vi "GetConfigFilePath.vi"(8 "error in (no error)":errorcluster caption="Fehler (Eingang, kein Fehler)", 10 "Main Vi Reference":refnum<vi>, 11 "ApplicationInititialisation Eingang":refnum<class "ApplicationInititialisation.lvclass"> caption="DNL_LabVIEW Object in") -> (0 "error out":errorcluster caption="Fehler (Ausgang)", 2 "Pfad":path, 3 "ApplicationInititialisation Ausgang":refnum<class "ApplicationInititialisation.lvclass"> caption="DNL_LabVIEW Object out")   [LabVIEW 2013, in "ApplicationInititialisation.lvclass"]
uses:
  ApplicationInititialisation.lvclass
panel:
  out "Ergebnis-String":string
  out "Applikation:Typ":T1(ring)
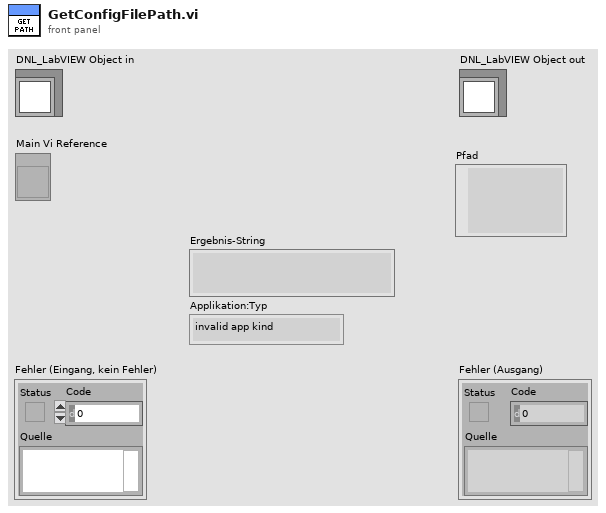
[diagram p1: front panel]
types:
  T1 = enum32{"invalid app kind", "Development System", "Run Time System", "Student Edition", "Embedded LabVIEW", "Evaluation", "Custom"}
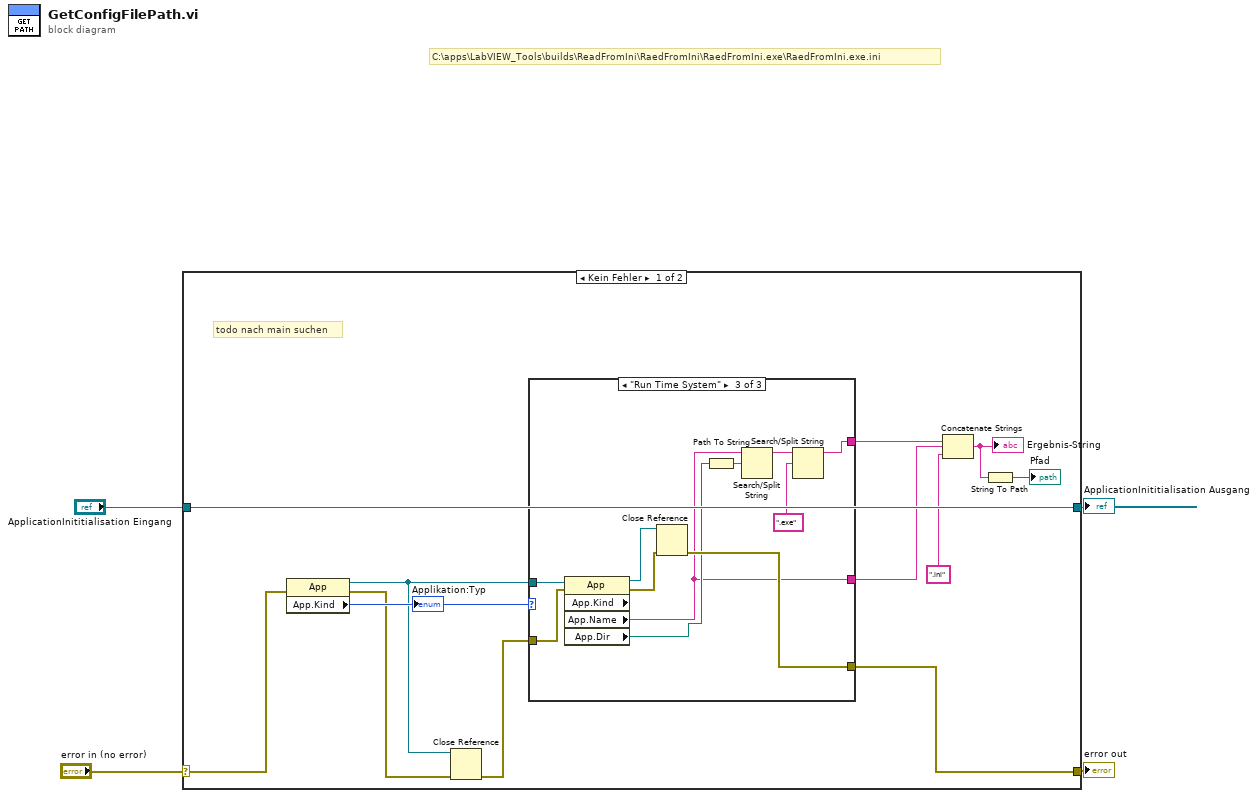
[diagram p0: block diagram]
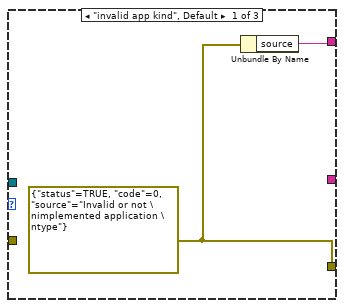
[diagram p2: hidden frame]
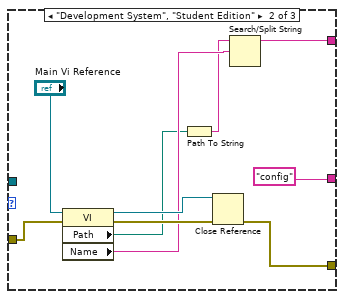
[diagram p3: hidden frame]
diagram:
  # "C:\\apps\\LabVIEW_Tools\\builds\\ReadFromIni\\RaedFromIni\\RaedFromIni.exe\\RaedFromIni.exe.ini"
  n1 = case shown="Kein Fehler" "error in (no error)" {
    selector: "error in (no error)" -> [w10 w41]
    tunnel: [w5 w41] -> w3
    tunnel: [w16 w40] -> w1
    tunnel: "ApplicationInititialisation Eingang" -> [w16 w40]
    frame No Error {
      # "todo nach main suchen"
      n2 = property class="App"(error in=w10) -> (reference out=w8:refnum<vi>, error out=w9:errorcluster, "App.Kind"=w15:T1)  [unwired: 1 in]
      "Applikation:Typ" <- w15
      n3 = Close Reference(reference=w8, error in (no error)=w9) -> (error out=w6:errorcluster)
      n4 = case shown="\"Run Time System\"" w15 {
        tunnel: [_ "config" w32] -> w11
        tunnel: w8 -> [_ _ w39]
        tunnel: [w18 w24 w36] -> w5
        tunnel: [w17 w20 w29] -> w7
        tunnel: w6 -> [_ w19 w35]
        frame "invalid app kind", Default {
          w18 = errorcluster {"status"=TRUE, "code"=0, "source"="Invalid or not \nimplemented application \ntype"} ("error out")
          n5 = Unbundle By Name(w18) -> ("source"=w17:string)
        }
        frame "Development System", "Student Edition" {
          n6 = property class="VI"(reference="Main Vi Reference", error in=w19) -> (reference out=w26:refnum<vi>, error out=w25:errorcluster, "Path"=w22:path, "Name"=w23:string)
          n7 = Path To String(path=w22) -> (string=w21:string)
          n8 = Close Reference(reference=w26, error in (no error)=w25) -> (error out=w24:errorcluster)
          n9 = Search/Split String(string=w21, search string/char (-)=w23) -> (substring before match=w20:string)  [unwired: 1 in, 2 out]
        }
        frame "Run Time System" {
          n10 = property class="App" props=["App.Kind", "App.Name", "App.Dir"](reference=w39, error in=w35) -> (reference out=w38:refnum<vi>, error out=w37:errorcluster, "App.Name"=w32:string, "App.Dir"=w34:path)  [unwired: 1 out]
          n11 = Close Reference(reference=w38, error in (no error)=w37) -> (error out=w36:errorcluster)
          n12 = Path To String(path=w34) -> (string=w33:string)
          n13 = Search/Split String(string=w32, search string/char (-)=w33) -> (substring before match=w31:string)  [unwired: 1 in, 2 out]
          n14 = Search/Split String(string=w31, search string/char (-)=".exe" ("Nach String/Zeichen suchen (-)")) -> (substring before match=w29:string)  [unwired: 1 in, 2 out]
        }
      }
      n15 = Concatenate Strings(w7, w11, ".ini") -> (w14:string)
      "Ergebnis-String" <- w14
      n16 = String To Path(string=w14) -> (path=→"Pfad":path)
    }
    frame Error {
    }
  }
  "error out" <- w3
  "ApplicationInititialisation Ausgang" <- w1
